vi "roic register finder.vi"(9 "String":string) -> (1 "match substring":string)   [LabVIEW 2018]
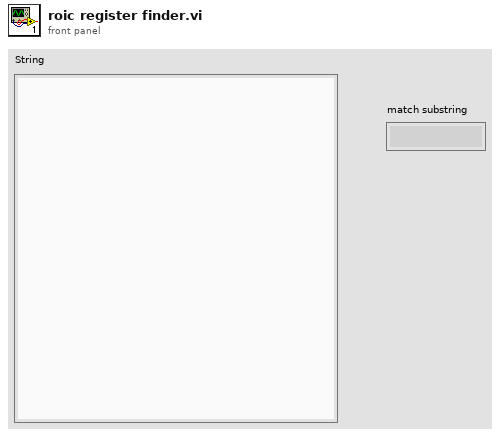
[diagram p1: front panel]
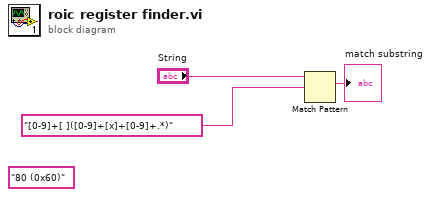
[diagram p0: block diagram]
diagram:
  (unwired) "80 (0x60)" ("regular expression")
  n1 = Match Pattern(string="String", regular expression="[0-9]+[ ]([0-9]+[x]+[0-9]+.*)") -> (match substring=→"match substring":string)  [unwired: 1 in, 3 out]
